vi "IP地址转换为数值.vi"(11 "IP地址":string="192.168.1.159") -> (0 "16进制数组":string[](array[string]), 2 "数组":u8[](array[numeric]), 3 "字符串数组":string[](array[string]))   [LabVIEW 2017]
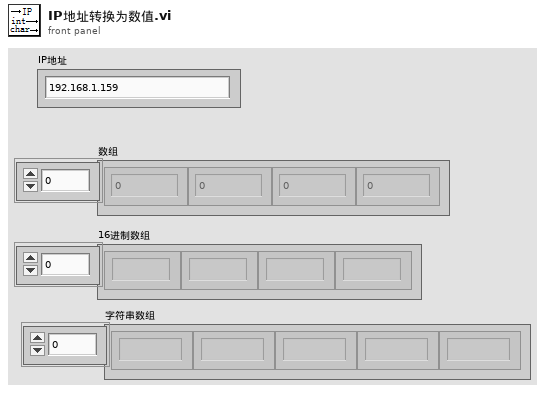
[diagram p1: front panel]
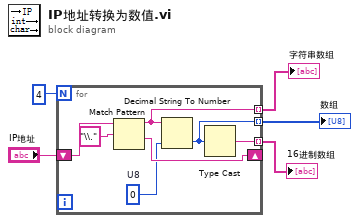
[diagram p0: block diagram]
diagram:
  n1 = for {
    N: 4 -> [_]
    shift-right: [w10] -> _
    shift-left: "IP地址" -> [w11]
    tunnel: [w8] -> w3 mode=indexing
    tunnel: [w7] -> w2 mode=indexing
    tunnel: [w6] -> w1 mode=indexing
    w9 = u8 0  # U8
    n2 = Match Pattern(string=w11, regular expression="\\." ("搜索字符串/字符(-)")) -> (before substring=w6:string, after substring=w10:string)  [unwired: 1 in, 2 out]
    n3 = Decimal String To Number(string=w6, default (0L)=w9) -> (number=w8:u8)  [unwired: 1 in, 1 out]
    n4 = Type Cast(x=w8) -> (*(type *) &x=w7:string)  [unwired: 1 in]
  }
  "数组" <- w3
  "16进制数组" <- w2
  "字符串数组" <- w1
